vi "Set_Configuration_Zurich.vi"(5 "Subscription 0":cluster{"path":string, "Channels":string[]}={"path"="/dev714/demods/0/sample.", "Channels"=["R", "Theta", "X", "Y", "AuxIn0", "AuxIn1", "Frequency", "Dio"]}, 6 "general settings double":cluster{"command":string, "value":dbl}[](array[cluster])=[{"command"="/dev714/oscs/0/freq", "value"=200000.0}, {"command"="/dev714/demods/0/order", "value"=8.0}, {"command"="/dev714/demods/0/timeconstant", "value"=9.57619476e-06}, {"command"="/dev714/demods/0/rate", "value"=115100.0}, {"command"="/dev714/demods/0/enable", "value"=1.0}, {"command"="/dev714/sigouts/0/amplitudes/6", "value"=1.0}, {"command"="/dev714/sigouts/0/enables/6", "value"=1.0}, {"command"="/dev714/sigouts/0/on", "value"=1.0}, {"command"="/dev714/oscs/1/freq", "value"=200000.0}, {"command"="/dev714/demods/3/order", "value"=8.0}, {"command"="/dev714/demods/3/timeconstant", "value"=9.57619e-06}, {"command"="/dev714/demods/3/rate", "value"=115100.0}, {"command"="/dev714/demods/3/enable", "value"=1.0}], 7 "data Acquisition Module double":cluster{"command":string, "value":dbl}[](array[cluster])=[{"command"="type", "value"=2.0}, {"command"="endless", "value"=0.0}, {"command"="duration", "value"=1.0}, {"command"="grid/mode", "value"=4.0}, {"command"="grid/cols", "value"=115100.0}, {"command"="bits", "value"=1.0}, {"command"="bitmask", "value"=1.0}, {"command"="edge", "value"=3.0}], 8 "error in":errorcluster, 9 "general settings string":cluster{"command":string, "value":string}[](array[cluster]), 10 "data Acquisition Module string":cluster{"command":string, "value":string}[](array[cluster])=[{"command"="device", "value"="dev714"}, {"command"="triggernode", "value"="/dev714/demods/0/sample.Dio"}, {"command"="", "value"=""}], 11 "Filename (.ini)":string="Config_Ver_1\\Zurich_params.ini") -> (0 "error out":errorcluster)   [LabVIEW 2021]
uses:
  <vilib>/Utility/config.llb/Write Key (String).vi
  <vilib>/Utility/config.llb/Write Key (Double).vi
  <vilib>/Utility/config.llb/NI_LVConfig.lvlib
panel:
  in  "Subscription 3":cluster{"path":string, "Channels":string[]}={"path"="/dev714/demods/3/sample.", "Channels"=["R", "Theta", "X", "Y", "AuxIn0", "AuxIn1", "Frequency", "Dio"]}
  # "sposób trigerowania"
  # "czas trwania"
  # "rozmieszczenie punktów (4- na siatce)"
  # "liczba punktów"
  # "triger na zboczu (3 - dowolnym)"
  # "częstotliwość modulacji/demodulacji na demodulatorze 0"
  # "rząd filtra LP na demodulatorze 0"
  # "stała czasowa (pasmo) filtra na dem 0"
  # "pasmo kolejki danych (Sa/s)"
  # "włacz kolejkę danych"
  # "amplituda wyj signal outp 1 (V)"
  # "włącz wzmocnienie na signal outp 1"
  # "włącz signal outp 1"
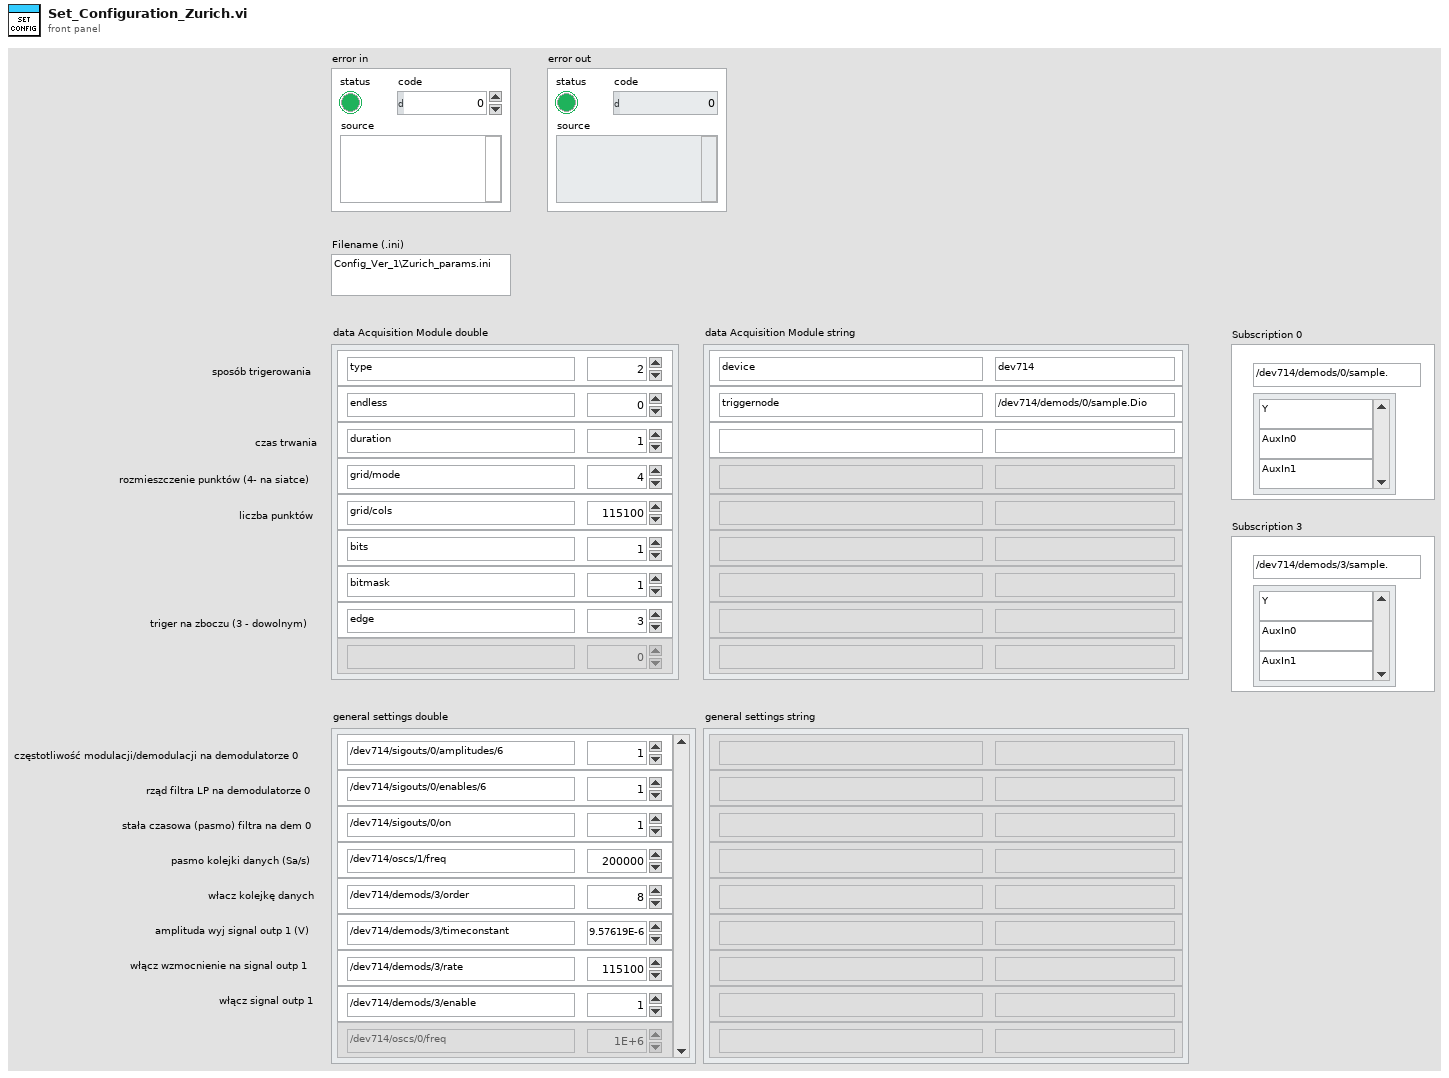
[diagram p1: front panel]
types:
  T1 = typedef "NI_LVConfig.lvlib/Config Data RefNum.ctl" = refnum<k1>
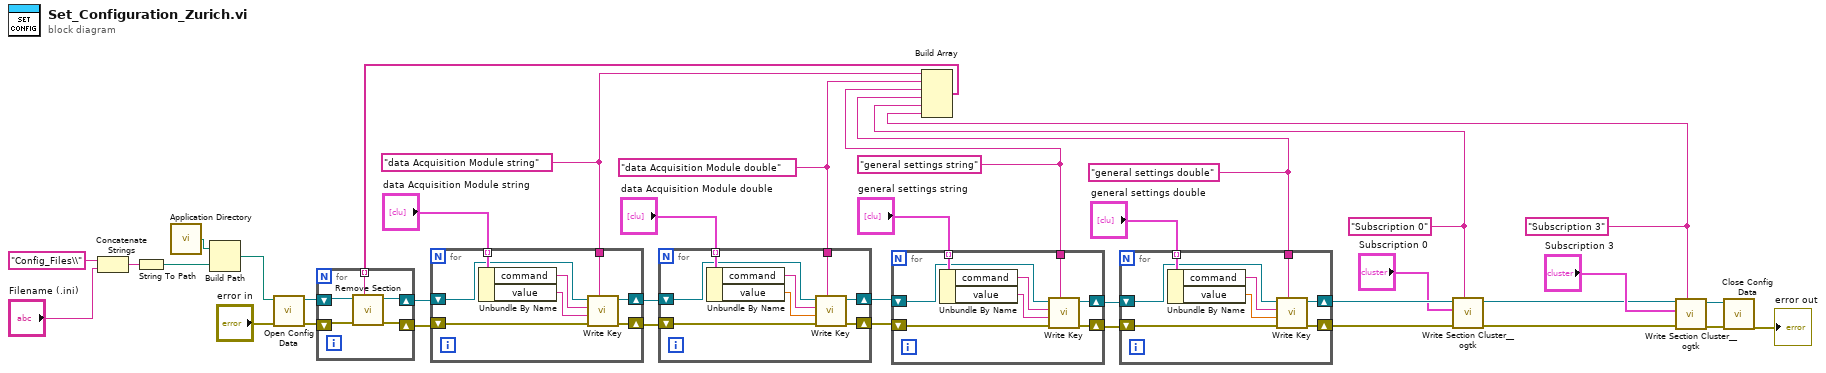
[diagram p0: block diagram]
diagram:
  w1 = "Subscription 3" ("section (optional)")
  w7 = "Subscription 0" ("section (optional)")
  w13 = "general settings double" ("section")
  w12 = "general settings string" ("section")
  w26 = "data Acquisition Module double" ("section")
  w25 = "data Acquisition Module string" ("section")
  n1 = Concatenate Strings("Config_Files\\" ("string"), "Filename (.ini)") -> (w36:string)
  n2 = String To Path(string=w36) -> (path=w33:path)
  n3 = call <vilib>:"Application Directory.vi"() -> ("Application Directory"=w31:path)
  n4 = Build Path(base path=w31, name or relative path=w33) -> (appended path=w32:path)
  n5 = call <vilib>:"Open Config Data.vi"("error in (no error)"="error in", "configuration file path"=w32) -> ("error out"=w24:errorcluster, "refnum"=w21:T1)  [unwired: 7 in, 1 out]
  n6 = Build Array(w25, w26, w12, w13, w7, w1) -> (w20:string[])
  n7 = for {
    shift-right: [w42] -> w22
    shift-left: w21 -> [w41]
    shift-right: [w39] -> w23
    shift-left: w24 -> [w40]
    tunnel: w20 -> [w38] mode=indexing
    n8 = call <vilib>:"Remove Section.vi"("section"=w38, "error in (no error)"=w40, "refnum"=w41) -> ("error out"=w39:errorcluster, "refnum out"=w42:T1)  [unwired: 6 in, 1 out]
  }
  n9 = for {
    shift-right: [w49] -> w29
    shift-left: w22 -> [w45]
    shift-right: [w50] -> w28
    shift-left: w23 -> [w44]
    tunnel: "data Acquisition Module string" -> [w48] mode=indexing
    tunnel: w25 -> [w43]
    n10 = Unbundle By Name(w48) -> ("command"=w46:string, "value"=w47:string)
    n11 = call-poly <vilib>:"Write Key.vi"("section"=w43, "error in (no error)"=w44, "value"=w47, "key"=w46, "refnum"=w45) -> ("error out"=w50:errorcluster, "refnum out"=w49:T1)  [unwired: 4 in, 1 out]
  }
  n12 = for {
    shift-right: [w57] -> w17
    shift-left: w29 -> [w53]
    shift-right: [w58] -> w16
    shift-left: w28 -> [w52]
    tunnel: "data Acquisition Module double" -> [w56] mode=indexing
    tunnel: w26 -> [w51]
    n13 = Unbundle By Name(w56) -> ("command"=w54:string, "value"=w55:dbl)
    n14 = call-poly <vilib>:"Write Key.vi"("section"=w51, "error in (no error)"=w52, "value"=w55, "key"=w54, "refnum"=w53) -> ("error out"=w58:errorcluster, "refnum out"=w57:T1)  [unwired: 4 in, 1 out]
  }
  n15 = for {
    shift-right: [w65] -> w18
    shift-left: w17 -> [w61]
    shift-right: [w66] -> w19
    shift-left: w16 -> [w60]
    tunnel: "general settings string" -> [w64] mode=indexing
    tunnel: w12 -> [w59]
    n16 = Unbundle By Name(w64) -> ("command"=w62:string, "value"=w63:string)
    n17 = call-poly <vilib>:"Write Key.vi"("section"=w59, "error in (no error)"=w60, "value"=w63, "key"=w62, "refnum"=w61) -> ("error out"=w66:errorcluster, "refnum out"=w65:T1)  [unwired: 4 in, 1 out]
  }
  n18 = for {
    shift-right: [w73] -> w10
    shift-left: w18 -> [w69]
    shift-right: [w74] -> w9
    shift-left: w19 -> [w68]
    tunnel: "general settings double" -> [w72] mode=indexing
    tunnel: w13 -> [w67]
    n19 = Unbundle By Name(w72) -> ("command"=w70:string, "value"=w71:dbl)
    n20 = call-poly <vilib>:"Write Key.vi"("section"=w67, "error in (no error)"=w68, "value"=w71, "key"=w70, "refnum"=w69) -> ("error out"=w74:errorcluster, "refnum out"=w73:T1)  [unwired: 4 in, 1 out]
  }
  n21 = call <userlib>:"Write Section Cluster__ogtk.vi"("section (optional)"=w7, "error in (no error)"=w9, "Section Formatted Cluster"="Subscription 0", "refnum"=w10) -> ("error out"=w4:errorcluster, "dup refnum"=w5:T1)  [unwired: 6 in]
  n22 = call <userlib>:"Write Section Cluster__ogtk.vi"("section (optional)"=w1, "error in (no error)"=w4, "Section Formatted Cluster"="Subscription 3", "refnum"=w5) -> ("error out"=w2:errorcluster, "dup refnum"=w3:T1)  [unwired: 6 in]
  n23 = call <vilib>:"Close Config Data.vi"("error in (no error)"=w2, "refnum"=w3) -> ("error out"=→"error out":errorcluster)  [unwired: 8 in, 1 out]
